vi "ReadFromTDMS.vi"(0 "文件名":string, 1 "通道名":string="声发射", 3 "时间长度":i32, 4 "起始时间":timestamp format="%<%H:%M:%S\n%x>T") -> (14 "数据":dbl[][](array[numeric]), 15 "时间":timestamp[](array[timestamp]), 16 "结束时间":timestamp format="%<%H:%M:%S\n%x>T", 19 "错误输出":errorcluster)   [LabVIEW 2014]
panel:
  out "数值":dbl
  out "组名称":string[](array[string])
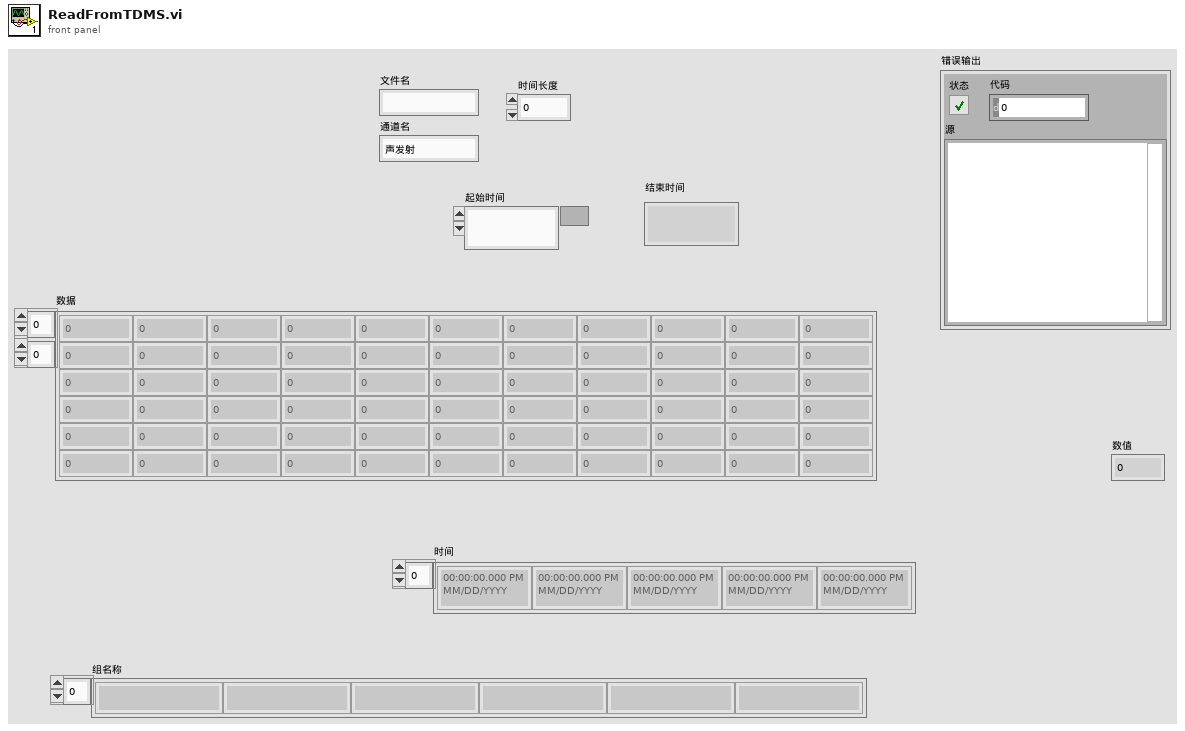
[diagram p1: front panel]
types:
  T1 = enum16{"open", "open or create", "create or replace", "create", "open (read-only)"}
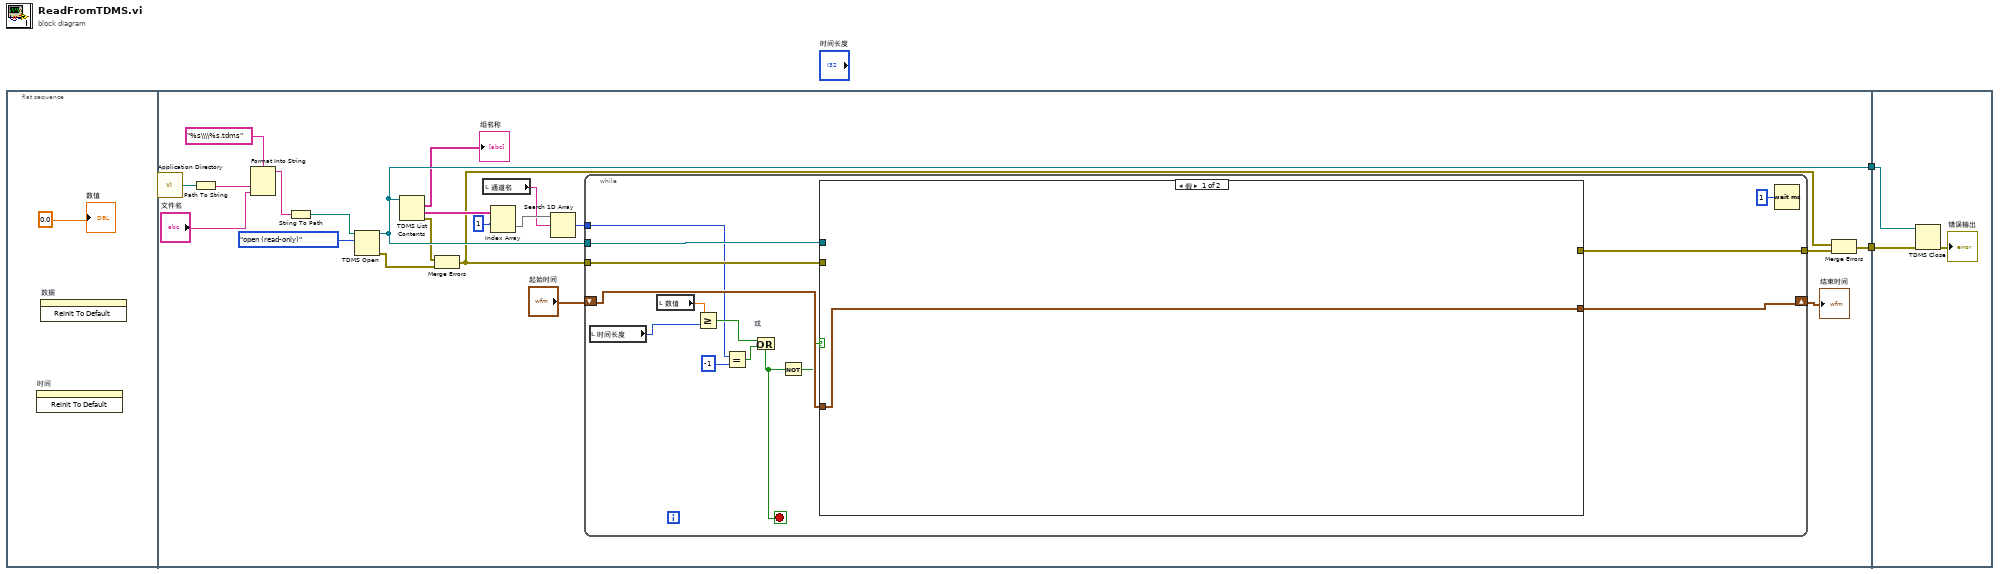
[diagram p0: block diagram]
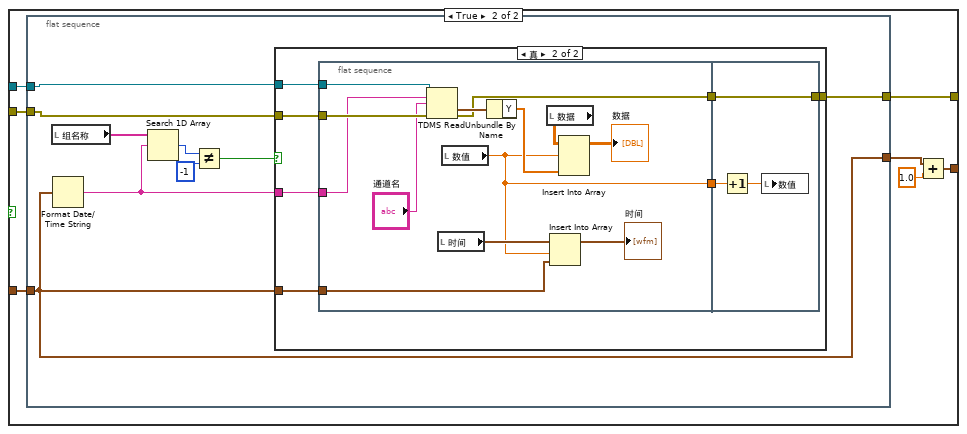
[diagram p2: hidden frame]
diagram:
  n1 = flat-sequence {
    tunnel: [w17] -> w2
    tunnel: [w7] -> w1
    tunnel: w2 -> [w80]
    tunnel: w1 -> [w79]
    frame #0 {
      n2 = invoke on="时间" class="Arr (严格)" method="Reinit To Default"() -> ()  [unwired: 3 in, 3 out]
      n3 = invoke on="数据" class="Arr (严格)" method="Reinit To Default"() -> ()  [unwired: 3 in, 3 out]
      "数值" <- 0.0
    }
    frame #1 {
      n4 = call <vilib>:"Application Directory.vi"() -> ("Application Directory"=w24:path)
      n5 = Path To String(path=w24) -> (string=w22:string)
      n6 = Format Into String(format string="%s\\\\%s.tdms", w22, "文件名") -> (resulting string=w21:string)  [unwired: 2 in, 1 out]
      n7 = String To Path(string=w21) -> (path=w18:path)
      n8 = TDMS Open(10:T1."open (read-only)" ("操作(0:open)"), 11:w18) -> (0:w10:errorcluster, 3:w17:refnum<k34>)  [unwired: 5 in]
      n9 = TDMS List Contents(7:w17) -> (0:w11:errorcluster, 1:w16:string[][], 2:→"组名称":string[])  [unwired: 2 in, 1 out]
      n10 = Merge Errors(w11, w10) -> (w8:errorcluster)
      n11 = local read "通道名"() -> (w13:string)
      n12 = Index Array(array=w16, index (row)=1 ("索引 (行)")) -> (element=w14:string[])  [unwired: 1 in]
      n13 = Search 1D Array(1D array=w14, element=w13) -> (index of element=w12:i32)  [unwired: 1 in]
      n14 = while {
        shift-right: [w26] -> w5
        shift-left: "起始时间" -> [w29]
        tunnel: w17 -> [w31]
        tunnel: w8 -> [w30]
        tunnel: w12 -> [w28]
        tunnel: [w37] -> w9
        stop <- w25 stop-if-true
        n15 = local read "时间长度"() -> (w36:i32)
        n16 = local read "数值"() -> (w35:dbl)
        n17 = Greater Or Equal?(x=w35, y=w36) -> (x >= y?=w34:bool)
        n18 = Equal?(x=w28, y=-1) -> (x = y?=w33:bool)
        n19 = Or "或"(x=w34, y=w33) -> (x .or. y?=w25:bool)
        n20 = Not(x=w25) -> (.not. x?=w27:bool)
        n21 = case shown="假" w27 {
          tunnel: w29 -> [w39 w46]
          tunnel: [_ w45] -> w37
          tunnel: w31 -> [_ w44]
          tunnel: w30 -> [_ w43]
          tunnel: [w39 w40] -> w26
          frame False {
          }
          frame True {
            n22 = flat-sequence {
              tunnel: [w50] -> w41
              tunnel: [w49] -> w45
              tunnel: w46 -> [w50]
              tunnel: w44 -> [w48]
              tunnel: w43 -> [w47]
              frame #0 {
                n23 = local read "组名称"() -> (w55:string[])
                n24 = Format Date/Time String(seconds (now)=w50) -> (date/time string=w54:string)  [unwired: 2 in]
                n25 = Search 1D Array(1D array=w55, element=w54) -> (index of element=w53:i32)  [unwired: 1 in]
                n26 = Not Equal?(x=w53, y=-1) -> (x != y?=w51:bool)
                n27 = case shown="真" w51 {
                  tunnel: w47 -> [_ w62]
                  tunnel: w48 -> [_ w61]
                  tunnel: w54 -> [_ w60]
                  tunnel: w50 -> [_ w58]
                  tunnel: [_ w56] -> w49
                  frame False {
                  }
                  frame True {
                    n28 = flat-sequence {
                      tunnel: w62 -> [w75]
                      tunnel: w61 -> [w73]
                      tunnel: w60 -> [w72]
                      tunnel: [w65] -> w59
                      tunnel: w58 -> [w64]
                      tunnel: [w63] -> w57
                      tunnel: w59 -> [w78]
                      tunnel: [w76] -> w56
                      tunnel: w57 -> [w76]
                      frame #0 {
                        n29 = TDMS Read(0:w73, 5:w72, 7:"通道名", 11:w75) -> (10:w68:waveform(dbl), 15:w63:errorcluster)  [unwired: 4 in, 4 out]
                        n30 = local read "时间"() -> (w66:timestamp[])
                        n31 = local read "数值"() -> (w65:dbl)
                        n32 = Unbundle By Name(w68) -> ("Y"=w69:dbl[])
                        n33 = local read "数据"() -> (w70:dbl[][])
                        n34 = Insert Into Array(array=w66, index=w65, new element=w64) -> (→"时间":timestamp[])
                        n35 = Insert Into Array(array=w70, index (row)=w65, new element=w69) -> (→"数据":dbl[][])  [unwired: 1 in]
                      }
                      frame #1 {
                        n36 = Increment(x=w78) -> (x+1=w77:dbl)
                        n37 = local write "数值"(w77) -> ()
                      }
                    }
                  }
                }
              }
            }
            n38 = Add(x=w41, y=1.0) -> (x+y=w40:timestamp)
          }
        }
        n39 = Wait (ms)(milliseconds to wait=u32 1 ("等待时间（毫秒）")) -> ()  [unwired: 1 out]
      }
      "结束时间" <- w5
      n40 = Merge Errors(w8, w9) -> (w7:errorcluster)
    }
    frame #2 {
      n41 = TDMS Close(8:w79, 11:w80) -> (0:→"错误输出":errorcluster)  [unwired: 1 out]
    }
  }
